vi "NI Get xxx Window name.vi"(8 "Error In":errorcluster) -> (0 "Error Out":errorcluster, 3 "X-Apps Name":string)   [LabVIEW 2018]
uses:
  LVWUtil32.dll
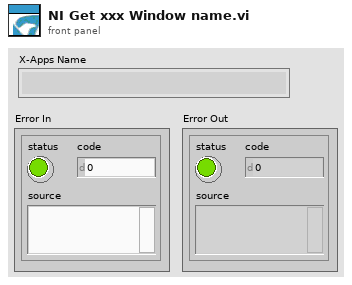
[diagram p1: front panel]
types:
  T1 = cluster{"number of windows":i32, "total names length":u32, "number of tasks found":i32, "window handles":u32[], "process ID":u32}
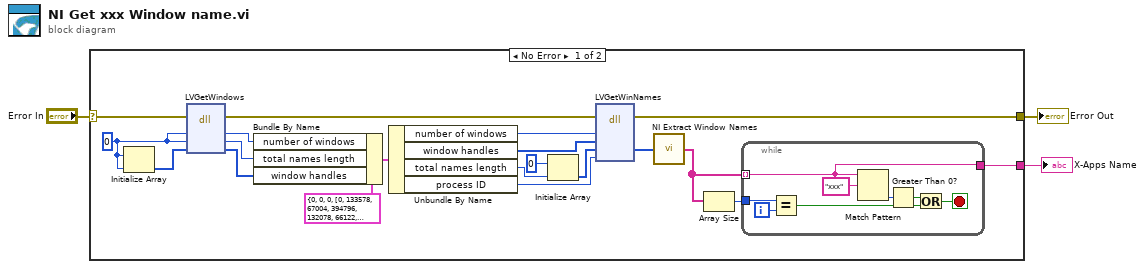
[diagram p0: block diagram]
diagram:
  n1 = case shown="No Error" "Error In" {
    selector: "Error In" -> [w4 w32]
    tunnel: [w8 w32] -> w3
    tunnel: [w5 _] -> w2
    frame No Error {
      w12 = u32 0
      n2 = Initialize Array(w12, w12) -> (w16:u32[])
      n3 = dll-call lib="C:/Users/John Gmitter/OneDrive - National Instruments/Projects/Harris FL/Manticore/Harris SW upgrades/Reference Management Server/Generic Reuse/Windows Utilities/LVWUtil32.dll" fn="LVGetWindows"(error in=w4, w12, w12, w16) -> (error out=w9:errorcluster, w13:i32, w14:u32, w15:u32[])  [unwired: 3 in, 1 out]
      n4 = Bundle By Name(cluster=T1 {"number of windows"=0, "total names length"=0, "number of tasks found"=0, "window handles"=[0, 133578, 67004, 394796, 132078, 66122, 66612, 41879366, 132718, 131234], "process ID"=0} ("window enumeration info in"), "number of windows"=w13, "total names length"=w14, "window handles"=w15) -> (w23:T1)
      n5 = Unbundle By Name(w23) -> ("number of windows"=w21:i32, "window handles"=w10:u32[], "total names length"=w11:u32, "process ID"=w19:u32)
      n6 = Initialize Array(u8 0, w11) -> (w20:u8[])
      n7 = dll-call lib="C:/Users/John Gmitter/OneDrive - National Instruments/Projects/Harris FL/Manticore/Harris SW upgrades/Reference Management Server/Generic Reuse/Windows Utilities/LVWUtil32.dll" fn="LVGetWinNames"(error in=w9, "numWin"=w21, w10, w20, "hInst"=w19) -> (error out=w8:errorcluster, w18:u8[])  [unwired: 6 in, 1 out]
      n8 = call "NI Extract Window Names.vi"("window names"=w18) -> ("application names"=w7:string[])
      n9 = Array Size(array=w7) -> (size(s)=w6:i32)
      n10 = while {
        tunnel: w7 -> [w24] mode=indexing
        tunnel: w6 -> [w30]
        tunnel: [w24] -> w5
        i -> [w29]
        stop <- w25 stop-if-true
        n11 = Equal?(x=w30, y=w29) -> (x = y?=w26:bool)
        n12 = Match Pattern(string=w24, regular expression="xxx") -> (offset past match=w28:i32)  [unwired: 1 in, 3 out]
        n13 = Greater Than 0?(x=w28) -> (x > 0?=w27:bool)
        n14 = Or(x=w27, y=w26) -> (x .or. y?=w25:bool)
      }
    }
    frame Error {
    }
  }
  "Error Out" <- w3
  "X-Apps Name" <- w2
